vi "VisualizeLog.vi"() -> ()   [LabVIEW 2018, in "Visualization.lvlib" / "VisualizeStatus.lvclass"]
doc: "This VI opens the error log on file and displays all errors that have been logged to file."
uses:
  VisualizeStatus.lvclass
  VisualizeBase/VisualizeBase_class/Requests/VisUserEventType.ctl
  <vilib>/event_ctls.llb/usereventprio.ctl
  <extravilib>/ChannelInstances/Tag-bool/Read With Abort.vi
  <extravilib>/ChannelInstances/Tag-bool/Write With Abort.vi
  <extravilib>/ChannelInstances/Tag-bool/Instantiate.vi
  <extravilib>/ChannelInstances/Tag-bool/EndpointRead.vi
  <vilib>/Utility/error.llb/Error Cluster From Error Code.vi
  <extravilib>/ChannelInstances/Tag-bool/Endpoint.vi
  <vilib>/ErrorRing/Error Ring.xnode
  VisualizeBase/VisualizeBase_class/VisualizeBase.lvclass
  <userlib>/NIST/NISTErrorLib/NISTErrorLib.lvlib
  <extravilib>/ChannelInstances/Tag-bool.lvlib
panel:
  in  "btnClearFile":bool
  in  "btnClear":bool
  out "error out":errorcluster
  in  "File Path Control":path
  out "Status Message":string
  in  "btnRefresh":bool
  in  "QueName":string="ErrorLogVisQue"
  out "ErrorArray":errorcluster[](array[cluster])
  in  "btnStop":bool
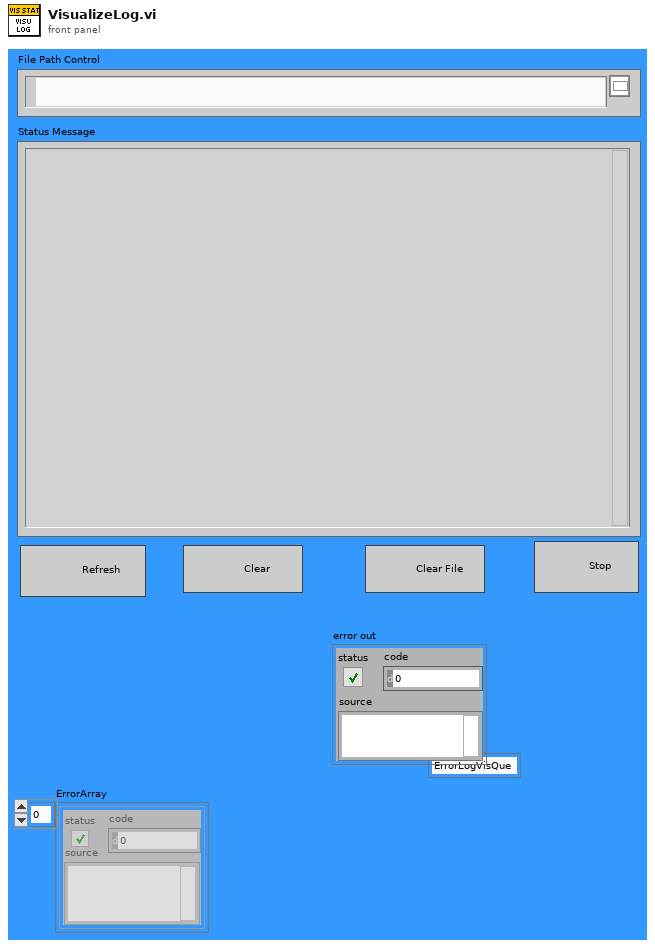
[diagram p1: front panel]
types:
  T1 = typedef "Visualization.lvlib/VisualizeBase.lvclass/VisRequestEvents.ctl" = cluster{"StopRequest":refnum<user-event>, "ResetRequest":refnum<user-event>, "FP Pop In or Out":refnum<user-event>}
  T2 = typedef "Visualization.lvlib/VisualizeBase.lvclass/VisUserEventType.ctl" = cluster{"BusIndex":i8, "Data":variant}
  T3 = typedef "usereventprio.ctl" = enum32{"high priority", "normal priority"}
  T4 = typedef "Tag-bool.lvlib/))Channel.ctl" = refnum<queue>
  T5 = enum16{"open", "replace", "create", "open or create", "replace or create", "replace or create with confirmation"}
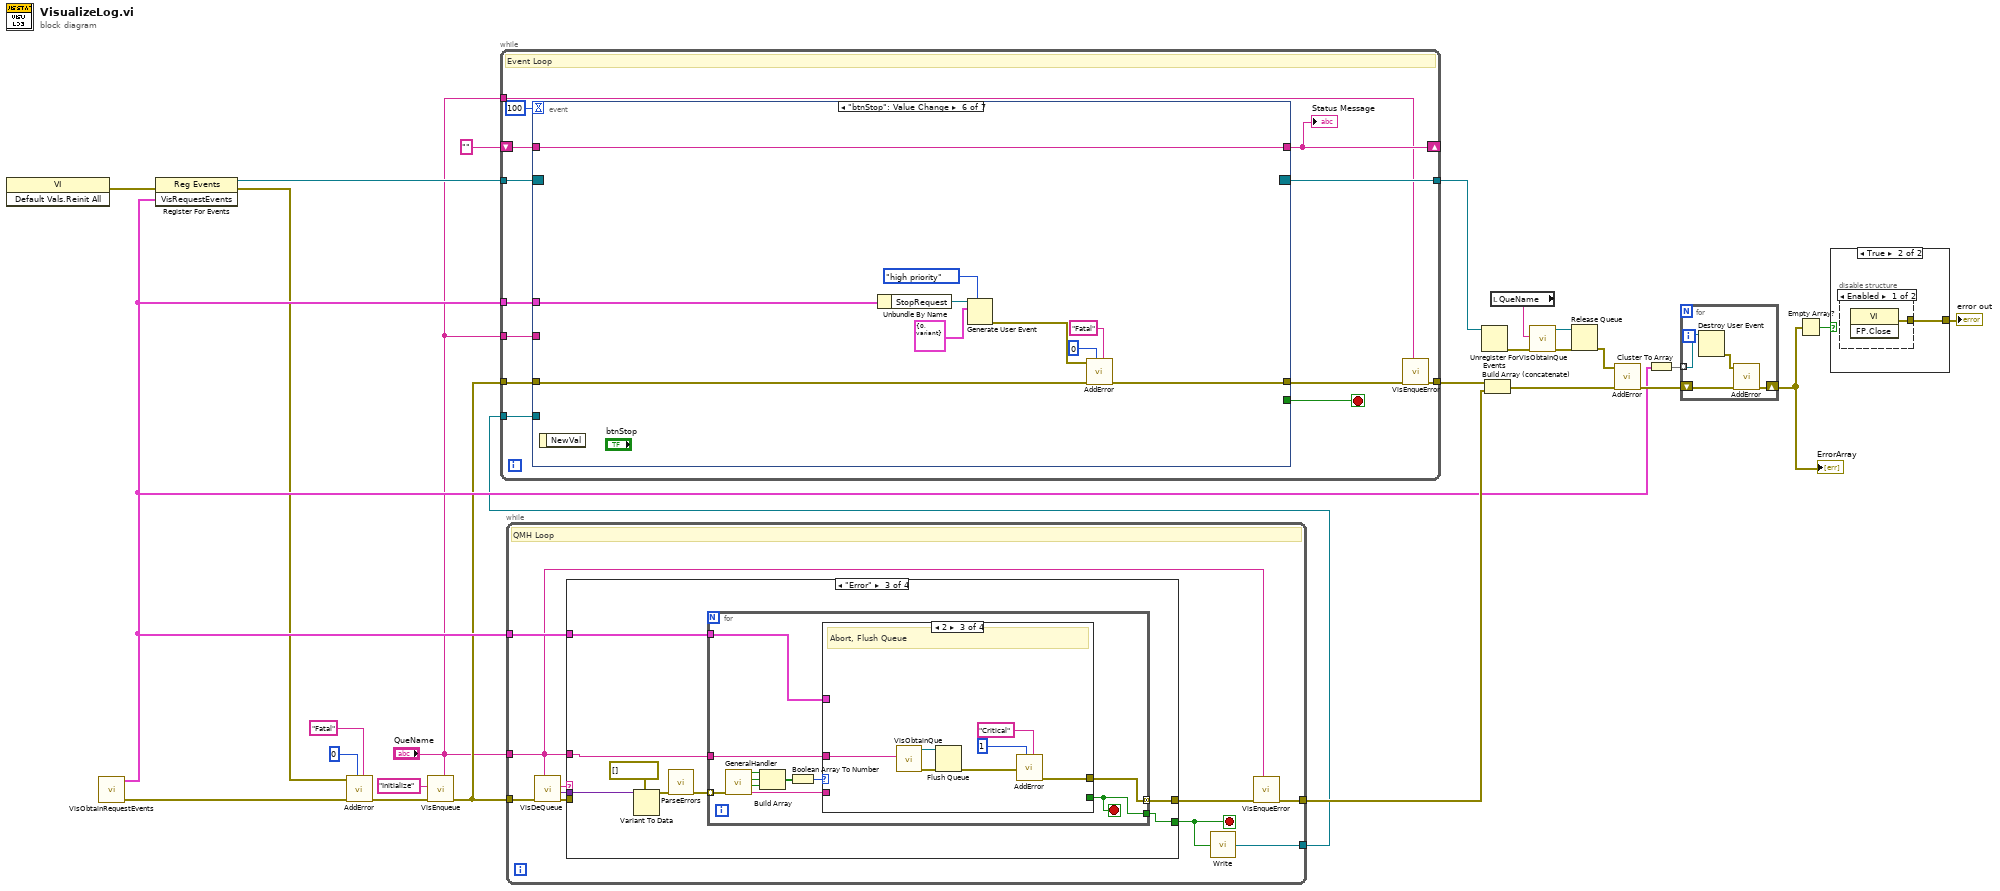
[diagram p0: block diagram]
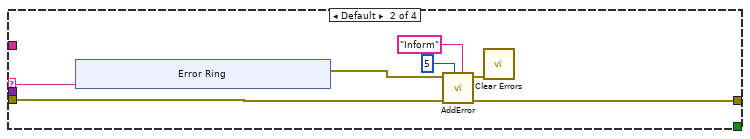
[diagram p3: hidden frame]
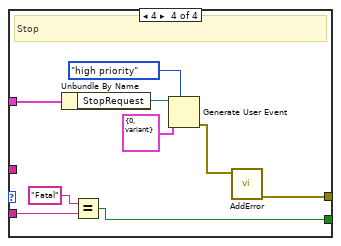
[diagram p6: hidden frame]
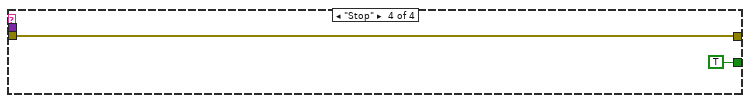
[diagram p7: hidden frame]
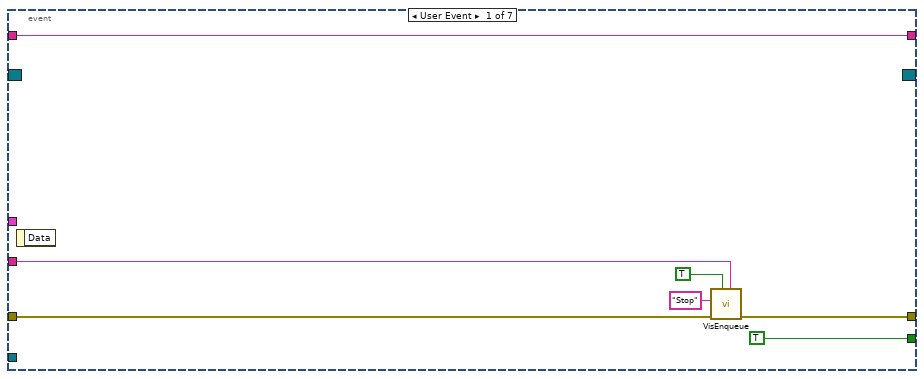
[diagram p8: hidden frame]
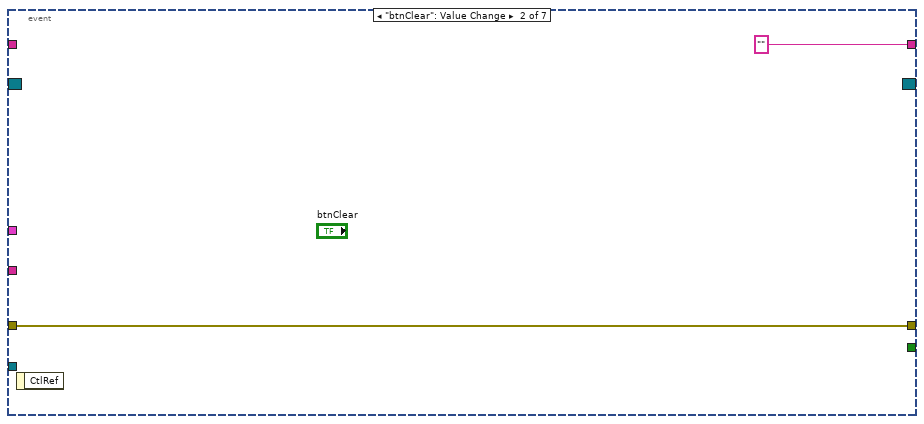
[diagram p9: hidden frame]
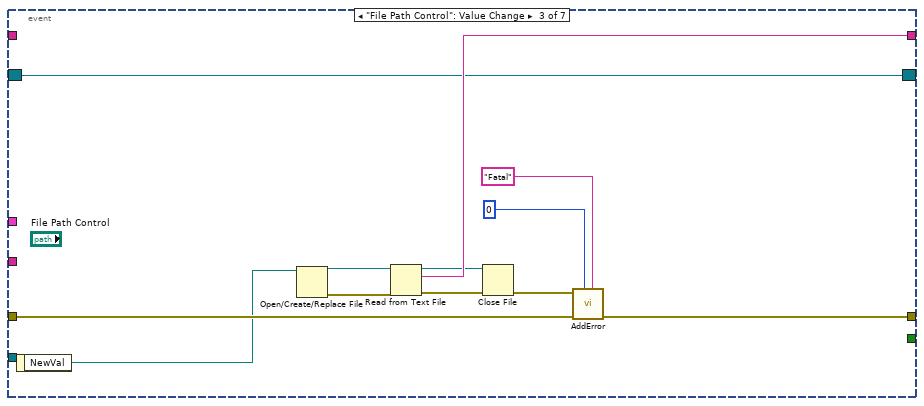
[diagram p10: hidden frame]
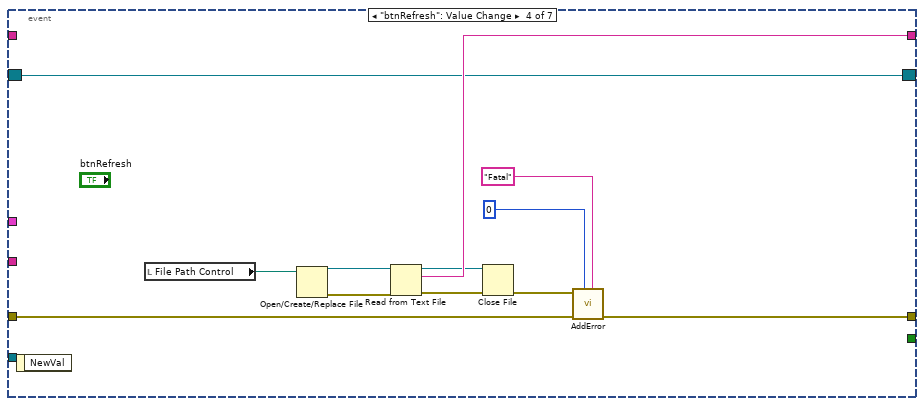
[diagram p11: hidden frame]
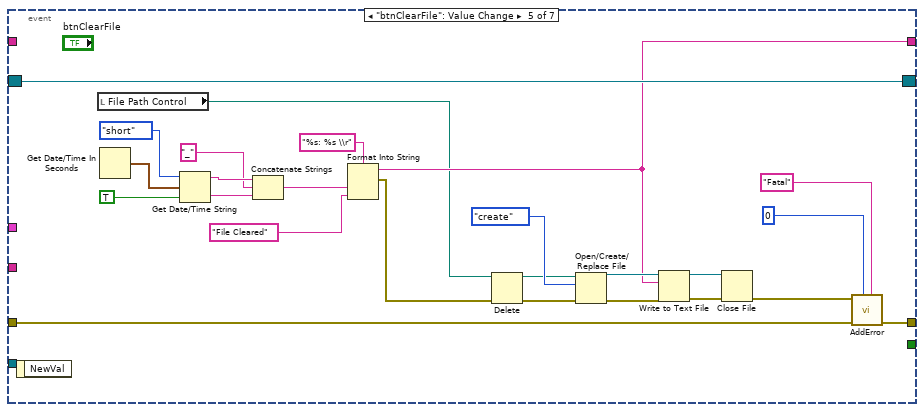
[diagram p12: hidden frame]
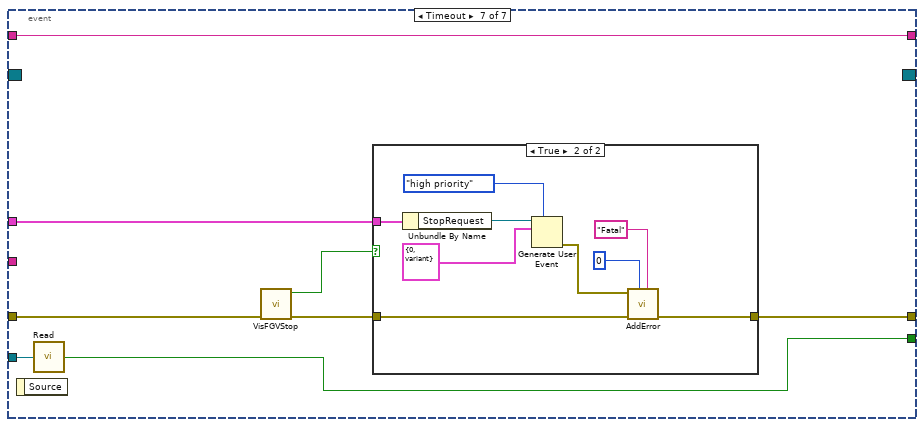
[diagram p13: hidden frame]
diagram:
  n1 = invoke class="VI" method="Default Vals.Reinit All"() -> (error out=w2:errorcluster)  [unwired: 3 in, 2 out]
  n2 = call "VisObtainRequestEvents.vi"() -> ("Error"=w26:errorcluster[], "VisRequestEvents"=w10:T1)  [unwired: 10 in]
  n3 = register-events(error in=w2, w10) -> (reference out=w11:refnum<event-registration>, error out=w9:errorcluster)  [unwired: 1 in]
  n4 = call <userlib>:"AddError.vi"("Severity"="Fatal", "Priority"=u8 0, "ErrorArray In"=w26, "error in (no error)"=w9) -> ("ErrorArray Out"=w12:errorcluster[])  [unwired: 6 in, 1 out]
  n5 = call "VisEnqueue.vi"("QueName"="QueName", "Error"=w12, "Message"="Initialize") -> ("Error"=w8:errorcluster[])  [unwired: 8 in]
  n6 = while {
    tunnel: w8 -> [w37]
    tunnel: [w31] -> w22
    tunnel: w10 -> [w30]
    tunnel: "QueName" -> [w29]
    tunnel: [w28] -> w1
    stop <- w32 stop-if-true
    # "QMH Loop"
    n7 = call "VisDeQueue.vi"("QueName"=w29, "Error"=w37) -> ("Error"=w34:errorcluster[], "Data"=w35:variant, "Message"=w36:string)  [unwired: 7 in]
    n8 = case shown="\"Error\"" w36 {
      selector: w36 -> [_ w45 _ _]
      tunnel: w35 -> [_ _ w60 _]
      tunnel: w34 -> [w38 w43 _ w88]
      tunnel: [w38 w42 w56 w88] -> w33
      tunnel: [_ _ w55 TRUE] -> w32
      tunnel: w30 -> [_ _ w54 _]
      tunnel: w29 -> [_ _ w53 _]
      frame "Initialize" {
      }
      frame Default {
        n9 = xnode "Error Ring"("parameter 0"=w45) -> ("error out"=w44:errorcluster)
        n10 = call <userlib>:"AddError.vi"("Severity"="Inform" ("String"), "Priority"=u8 5, "ErrorArray In"=w43, "error in (no error)"=w44) -> ("ErrorArray Out"=w42:errorcluster[], "error out"=w41:errorcluster)  [unwired: 6 in]
        n11 = call <vilib>:"Clear Errors.vi"("error in (no error)"=w41) -> ()  [unwired: 5 in, 2 out]
      }
      frame "Error" {
        n12 = Variant To Data(type=errorcluster[] [], Variant=w60) -> (data=w58:errorcluster[])  [unwired: 1 in, 1 out]
        n13 = call <userlib>:"ParseErrors.vi"("ErrorArray"=w58) -> ("ErrorArray"=w57:errorcluster[])  [unwired: 8 in, 2 out]
        n14 = for {
          tunnel: w57 -> [w71] mode=indexing
          tunnel: [w65] -> w56 mode=concatenating
          tunnel: [w63] -> w55
          tunnel: w54 -> [w62]
          tunnel: w53 -> [w61]
          stop <- w63 stop-if-true
          n15 = call <userlib>:"GeneralHandler.vi"("error in (no error)"=w71) -> ("Severity"=w64:string, "Stop"=w68:bool, "Abort"=w69:bool, "Continue"=w70:bool)  [unwired: 6 in, 1 out]
          n16 = Build Array(w70, w69, w68) -> (w67:bool[])
          n17 = Boolean Array To Number(Boolean array=w67) -> (number=w66:u32)
          n18 = case shown="2" w66 {
            tunnel: [_ _ w76 w86] -> w65
            tunnel: w64 -> [_ _ _ w82]
            tunnel: [_ _ _ w80] -> w63
            tunnel: w62 -> [_ _ _ w79]
            tunnel: w61 -> [_ _ w72 _]
            frame 0, Default {
              # "No Dialog"
            }
            frame 1 {
              # "Continue"
            }
            frame 2 {
              # "Abort, Flush Queue"
              n19 = call "VisObtainQue.vi"("QueName"=w72) -> ("error out"=w78:errorcluster, "queue out"=w77:refnum<queue>)  [unwired: 9 in]
              n20 = Flush Queue(queue=w77, error in (no error)=w78) -> (error out=w75:errorcluster)  [unwired: 2 out]
              n21 = call <userlib>:"AddError.vi"("Severity"="Critical" ("String"), "Priority"=u8 1, "error in (no error)"=w75) -> ("ErrorArray Out"=w76:errorcluster[])  [unwired: 7 in, 1 out]
            }
            frame 4 {
              # "Stop"
              n22 = Unbundle By Name(w79) -> ("StopRequest"=w87:refnum<user-event>)
              n23 = Equal?(x="Fatal", y=w82) -> (x = y?=w80:bool)
              n24 = Generate User Event(priority (normal)=usereventprio."high priority", user event=w87, event data cluster=T2 {"BusIndex"=0, "Data"=variant} ("event data")) -> (error out=w85:errorcluster)  [unwired: 1 in, 1 out]
              n25 = call <userlib>:"AddError.vi"("error in (no error)"=w85) -> ("ErrorArray Out"=w86:errorcluster[])  [unwired: 9 in, 1 out]
            }
          }
        }
      }
      frame "Stop" {
      }
    }
    n26 = call <extravilib>:"Write.vi"("element"=w32) -> ("channel"=w28:T4)  [unwired: 1 out]
    n27 = call "VisEnqueError.vi"("QueName"=w29, "Error"=w33) -> ("Error"=w31:errorcluster[])  [unwired: 9 in]
  }
  n28 = while {
    tunnel: w11 -> [w102]
    tunnel: [w99] -> w23
    tunnel: [w98] -> w25
    tunnel: w10 -> [w97]
    shift-right: [w94] -> _
    shift-left: "" -> [w96]
    tunnel: w8 -> [w95]
    tunnel: "QueName" -> [w93]
    tunnel: "QueName" -> [w92]
    tunnel: w1 -> [w90]
    stop <- w101 stop-if-true
    # "Event Loop"
    n29 = event shown="[5] \"btnStop\": Value Change" {
      selector: w102 -> [_ _ w112 w125 w151 _ _]
      dyn-events: [_ _ w112 w125 w151 _ _] -> w98
      timeout: 100 -> [_ _ _ _ _ _ _]
      tunnel: [TRUE _ _ _ _ _ w171] -> w101
      tunnel: [w108 w110 w117 w129 w155 w168 w178] -> w100
      tunnel: w97 -> [_ _ _ _ _ w163 w177]
      tunnel: [w103 "" w121 w133 w141 w161 w176] -> w94
      tunnel: w96 -> [w103 _ _ _ _ w161 w176]
      tunnel: w95 -> [w104 w110 w118 w130 w156 w162 w174]
      tunnel: w92 -> [w105 _ _ _ _ _ _]
      tunnel: w90 -> [_ _ _ _ _ _ w172]
      event User Event {
        n30 = event-data() -> ()  [unwired: 1 in, 1 out]
        n31 = call "VisEnqueue.vi"("QueName"=w105, "Priority? (F)"=TRUE, "Error"=w104, "Message"="Stop") -> ("Error"=w108:errorcluster[])  [unwired: 7 in]
      }
      event "btnClear": Value Change {
        n32 = event-data() -> ()  [unwired: 1 in, 1 out]
      }
      event "File Path Control": Value Change {
        n33 = event-data() -> ("NewVal"=w113:path)  [unwired: 1 in]
        n34 = Open/Create/Replace File(file path (use dialog)=w113) -> (refnum out=w122:refnum<file>, error out=w123:errorcluster)  [unwired: 5 in, 1 out]
        n35 = Read from Text File(file (use dialog)=w122, error in=w123) -> (refnum out=w119:refnum<file>, text=w121:string, error out=w120:errorcluster)  [unwired: 2 in, 1 out]
        n36 = Close File(refnum=w119, error in=w120) -> (error out=w116:errorcluster)  [unwired: 1 out]
        n37 = call <userlib>:"AddError.vi"("Severity"="Fatal", "Priority"=u8 0, "ErrorArray In"=w118, "error in (no error)"=w116) -> ("ErrorArray Out"=w117:errorcluster[])  [unwired: 6 in, 1 out]
      }
      event "btnRefresh": Value Change {
        n38 = event-data() -> ()  [unwired: 1 in, 1 out]
        n39 = local read "File Path Control"() -> (w124:path)
        n40 = Open/Create/Replace File(file path (use dialog)=w124) -> (refnum out=w134:refnum<file>, error out=w135:errorcluster)  [unwired: 5 in, 1 out]
        n41 = Read from Text File(file (use dialog)=w134, error in=w135) -> (refnum out=w131:refnum<file>, text=w133:string, error out=w132:errorcluster)  [unwired: 2 in, 1 out]
        n42 = Close File(refnum=w131, error in=w132) -> (error out=w128:errorcluster)  [unwired: 1 out]
        n43 = call <userlib>:"AddError.vi"("Severity"="Fatal", "Priority"=u8 0, "ErrorArray In"=w130, "error in (no error)"=w128) -> ("ErrorArray Out"=w129:errorcluster[])  [unwired: 6 in, 1 out]
      }
      event "btnClearFile": Value Change {
        n44 = event-data() -> ()  [unwired: 1 in, 1 out]
        n45 = local read "File Path Control"() -> (w139:path)
        n46 = Get Date/Time In Seconds() -> (seconds since 1Jan1904=w150:timestamp)
        n47 = Get Date/Time String(date format (0)=enum16{"short", "long", "abbreviated"}."short", seconds (now)=w150, want seconds? (F)=TRUE) -> (date string=w148:string, time string=w149:string)
        n48 = Concatenate Strings(w148, "_" ("string"), w149) -> (w147:string)
        n49 = Format Into String(format string="%s: %s \\r", w147, "File Cleared" ("Severity")) -> (resulting string=w141:string, error out=w138:errorcluster)  [unwired: 2 in]
        n50 = Delete(path (use dialog)=w139, error in=w138) -> (deleted path=w136:path, error out=w137:errorcluster)  [unwired: 3 in, 1 out]
        n51 = Open/Create/Replace File(file path (use dialog)=w136, error in=w137, operation (0:open)=T5."create") -> (refnum out=w159:refnum<file>, error out=w160:errorcluster)  [unwired: 3 in, 1 out]
        n52 = Write to Text File(file (use dialog)=w159, text=w141, error in=w160) -> (refnum out=w157:refnum<file>, error out=w158:errorcluster)  [unwired: 1 in, 1 out]
        n53 = Close File(refnum=w157, error in=w158) -> (error out=w154:errorcluster)  [unwired: 1 out]
        n54 = call <userlib>:"AddError.vi"("Severity"="Fatal", "Priority"=u8 0, "ErrorArray In"=w156, "error in (no error)"=w154) -> ("ErrorArray Out"=w155:errorcluster[])  [unwired: 6 in, 1 out]
      }
      event "btnStop": Value Change {
        n55 = event-data() -> ()  [unwired: 1 in, 1 out]
        n56 = Unbundle By Name(w163) -> ("StopRequest"=w169:refnum<user-event>)
        n57 = Generate User Event(priority (normal)=usereventprio."high priority", user event=w169, event data cluster=T2 {"BusIndex"=0, "Data"=variant} ("event data")) -> (error out=w170:errorcluster)  [unwired: 1 in, 1 out]
        n58 = call <userlib>:"AddError.vi"("Severity"="Fatal" ("String"), "Priority"=u8 0, "ErrorArray In"=w162, "error in (no error)"=w170) -> ("ErrorArray Out"=w168:errorcluster[])  [unwired: 6 in, 1 out]
      }
      event Timeout {
        n59 = event-data() -> ()  [unwired: 1 in, 1 out]
        n60 = call <extravilib>:"Read.vi"("channel"=w172) -> ("element"=w171:bool)  [unwired: 1 in, 1 out]
        n61 = call "VisFGVStop.vi"("Error In"=w174) -> ("Error Out"=w173:errorcluster[], "Value"=w175:bool)  [unwired: 9 in]
        n62 = case shown="True" w175 {
          tunnel: [w179 w186] -> w178
          tunnel: w177 -> [_ w181]
          tunnel: w173 -> [w179 w180]
          frame False {
          }
          frame True {
            n63 = Unbundle By Name(w181) -> ("StopRequest"=w187:refnum<user-event>)
            n64 = Generate User Event(priority (normal)=usereventprio."high priority", user event=w187, event data cluster=T2 {"BusIndex"=0, "Data"=variant} ("event data")) -> (error out=w188:errorcluster)  [unwired: 1 in, 1 out]
            n65 = call <userlib>:"AddError.vi"("Severity"="Fatal" ("String"), "Priority"=u8 0, "ErrorArray In"=w180, "error in (no error)"=w188) -> ("ErrorArray Out"=w186:errorcluster[])  [unwired: 6 in, 1 out]
          }
        }
      }
    }
    "Status Message" <- w94
    n66 = call "VisEnqueError.vi"("QueName"=w93, "Error"=w100) -> ("Error"=w99:errorcluster[])  [unwired: 9 in]
  }
  n67 = Unregister For Events(event registration refnum=w25) -> (error out=w21:errorcluster)  [unwired: 1 in]
  n68 = Build Array (concatenate)(w23, w22) -> (w19:errorcluster[])
  n69 = local read "QueName"() -> (w20:string)
  n70 = call "VisObtainQue.vi"("error in (no error)"=w21, "QueName"=w20) -> ("error out"=w18:errorcluster, "queue out"=w17:refnum<queue>)  [unwired: 8 in]
  n71 = Release Queue(queue=w17, error in (no error)=w18) -> (error out=w16:errorcluster)  [unwired: 1 in, 2 out]
  n72 = call <userlib>:"AddError.vi"("ErrorArray In"=w19, "error in (no error)"=w16) -> ("ErrorArray Out"=w15:errorcluster[])  [unwired: 8 in, 1 out]
  n73 = Cluster To Array(cluster=w10) -> (array=w24:refnum<user-event>[])
  n74 = for {
    tunnel: w24 -> [w192] mode=indexing
    shift-right: [w191] -> w14
    shift-left: w15 -> [w190]
    n75 = Destroy User Event(user event=w192) -> (error out=w189:errorcluster)  [unwired: 1 in]
    n76 = call <userlib>:"AddError.vi"("ErrorArray In"=w190, "error in (no error)"=w189) -> ("ErrorArray Out"=w191:errorcluster[])  [unwired: 8 in, 1 out]
  }
  "ErrorArray" <- w14
  n77 = Empty Array?(array=w14) -> (empty?=w13:bool)
  n78 = case shown="True" w13 {
    tunnel: [_ w193] -> w3
    frame False {
    }
    frame True {
      n79 = disable-structure shown="Enabled" {
        disable-tunnel: [w194 _] -> w193
        frame Enabled {
          n80 = invoke class="VI" method="FP.Close"() -> (error out=w194:errorcluster)  [unwired: 3 in, 2 out]
        }
        frame Disabled {
        }
      }
    }
  }
  "error out" <- w3
